vi "Sub_time_to_time.vi"(1 "Time":string) -> (0 "Time hh::mm":string)   [LabVIEW 2023]
doc: "Converts string of time hh::mm::ss to hh::mm"
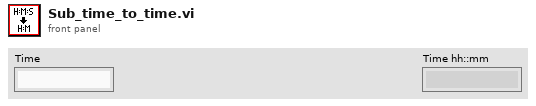
[diagram p1: front panel]
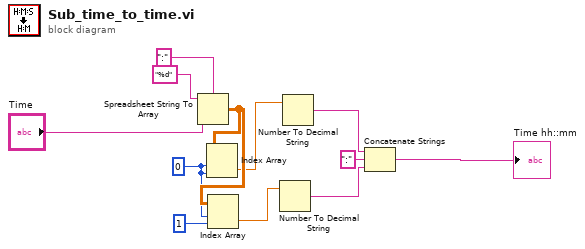
[diagram p0: block diagram]
diagram:
  w10 = 0 ("index (row)")
  n1 = Spreadsheet String To Array(delimiter (Tab)=":", format string="%d", spreadsheet string="Time") -> (array=w11:dbl[][])  [unwired: 1 in]
  n2 = Index Array(array=w11, index (row)=w10, index (col)=w10) -> (element=w6:dbl)
  n3 = Index Array(array=w11, index (row)=w10, index (col)=1 ("disabled index (col)")) -> (element=w2:dbl)
  n4 = Number To Decimal String(number=w2) -> (decimal integer string=w7:string)  [unwired: 1 in]
  n5 = Number To Decimal String(number=w6) -> (decimal integer string=w8:string)  [unwired: 1 in]
  n6 = Concatenate Strings(w8, ":" ("string"), w7) -> (→"Time hh::mm":string)
